vi "Read Coils.vi"(7 "unit ID":u8, 8 "error in":errorcluster, 9 "number of inputs":u16, 10 "starting address":u16, 11 "Modbus slave in":refnum<class "Modbus Slave.lvclass">) -> (0 "error out":errorcluster, 2 "coils":bool[](array[boolean]), 3 "Modbus slave out":refnum<class "Modbus Slave.lvclass">)   [LabVIEW 2013, in "Modbus Library - Advance.lvlib" / "Modbus Slave.lvclass"]
doc: "Reads <B>number of inputs</B> coils starting at <B>starting address</B> from the device."
uses:
  Modbus Slave.lvclass
  Modbus Slave.lvclass/Modbus Slave.ctl
  Standard Data Model/Standard Data Model.lvclass
  Super Data Model/Super Data Model.lvclass
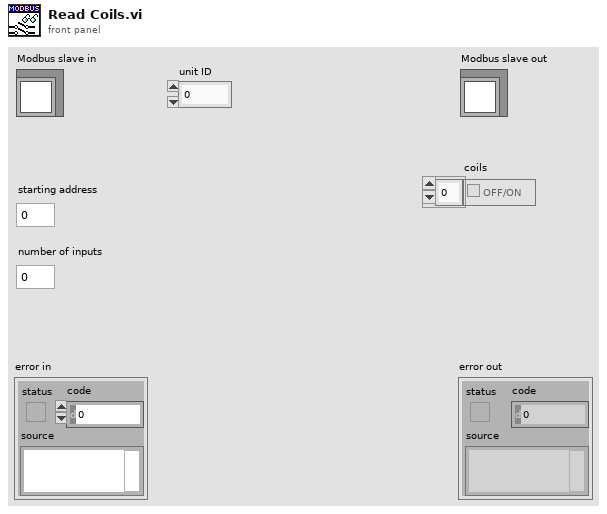
[diagram p1: front panel]
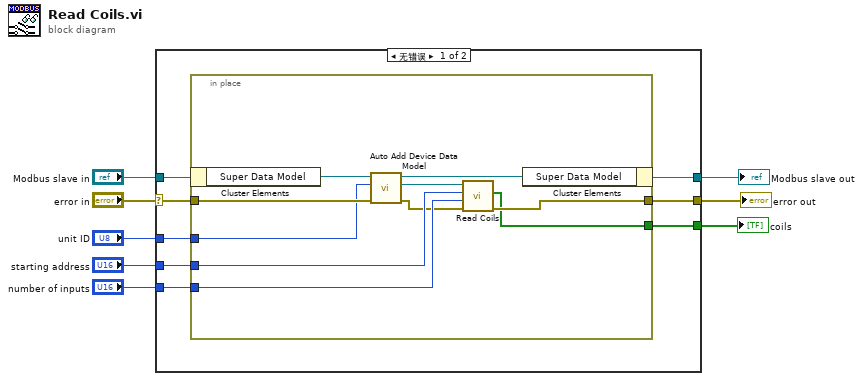
[diagram p0: block diagram]
diagram:
  n1 = case shown="无错误" "error in" {
    selector: "error in" -> [w14 w28]
    tunnel: [w11 w28] -> w1
    tunnel: "Modbus slave in" -> [w12 w27]
    tunnel: "number of inputs" -> [w16 _]
    tunnel: "starting address" -> [w15 _]
    tunnel: [w13 w27] -> w2
    tunnel: "unit ID" -> [w10 _]
    tunnel: [w9 _] -> w3
    frame No Error {
      n2 = in-place {
        in-place-border: w16 -> [w26]
        in-place-border: w15 -> [w25]
        in-place-border: w14 -> [w22]
        in-place-border: [w24] -> w11
        in-place-border: w10 -> [w21]
        in-place-border: [w19] -> w9
        n3 = in-place-cluster #1(w12) -> ("Super Data Model"=w23:refnum<class "Super Data Model.lvclass">)
        n4 = call "Auto Add Device Data Model.vi"("error in"=w22, "unit ID"=w21, "Super Data Model in"=w23) -> ("error out"=w17:errorcluster, "device data model"=w18:refnum<class "Standard Data Model.lvclass">, "Super Data Model out"=w20:refnum<class "Super Data Model.lvclass">)  [unwired: 6 in]
        n5 = call-dynamic "Read Coils.vi"("error in"=w17, "number of coils"=w26, "starting address"=w25, "device data model in"=w18) -> ("error out"=w24:errorcluster, "data"=w19:bool[])  [unwired: 5 in, 1 out]
        n6 = in-place-cluster #1("Super Data Model"=w20) -> (w13:refnum<class "Modbus Slave.lvclass">)
      }
    }
    frame Error {
    }
  }
  "error out" <- w1
  "Modbus slave out" <- w2
  "coils" <- w3
